vi "XY Graph Get Plots Metadata.vi"(8 "Error In":errorcluster, 11 "XYGraph Ref":T1) -> (0 "Error Out":errorcluster, 1 "Plot Metadata Found?":bool, 2 "Plot Metadata":variant[](array[variant]), 3 "XYGraph Ref (dup)":T1)   [LabVIEW 2021, in "XY Graph Add-Ons.lvlib"]
uses:
  XY Graph Add-Ons.lvlib
  XY Graph Refnum.ctl
  XY Graph Property Tag List.ctl
  <vilib>/UserTags/UserTags.lvlib
panel:
  # "see the License on the block diagram (Ctrl+E or Window:Show Block Diagram)"
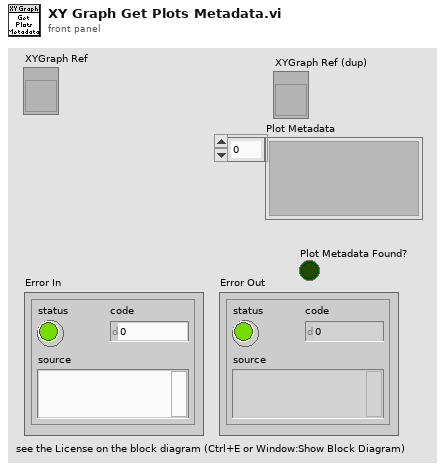
[diagram p1: front panel]
types:
  T1 = typedef "XY Graph Add-Ons.lvlib/XY Graph Refnum.ctl" = refnum<vi>
  T2 = typedef "XY Graph Add-Ons.lvlib/XY Graph Property Tag List.ctl" = enum16{"Max Legend Size", "Preserved Plots", "XScales.GridColors", "YScales.GridColors", "TipStrip String", "TipStrip Visible", "Tool Panels Visibility", "Plot Metadata"}
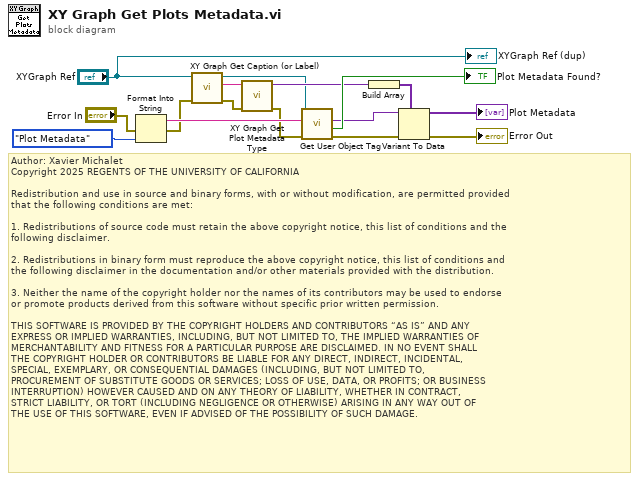
[diagram p0: block diagram]
diagram:
  # "Author: Xavier Michalet\nCopyright 2025 REGENTS OF THE UNIVERSITY OF CALIFORNIA\n\nRedistribution and use in source and binary forms, with or without modification, are permitted provided\nthat the following conditions are met:\n\n1. Redistributions of source code must retain the above copyright notice, this list of conditions and the\nfollowing disclaimer.\n\n2. Redistributions in binary form must reproduce the above copyright notice, this list of conditions and\nthe following disclaimer in the documentation and/or other materials provided with the distribution.\n\n3. Neither the name of the copyright holder nor the names of its contributors may be used to endorse \nor promote products derived from this software without specific prior written permission.\n\nTHIS SOFTWARE IS PROVIDED BY THE COPYRIGHT HOLDERS AND CONTRIBUTORS “AS IS” AND ANY \nEXPRESS OR IMPLIED WARRANTIES, INCLUDING, BUT NOT LIMITED TO, THE IMPLIED WARRANTIES OF\nMERCHANTABILITY AND FITNESS FOR A PARTICULAR PURPOSE ARE DISCLAIMED. IN NO EVENT SHALL\nTHE COPYRIGHT HOLDER OR CONTRIBUTORS BE LIABLE FOR ANY DIRECT, INDIRECT, INCIDENTAL, \nSPECIAL, EXEMPLARY, OR CONSEQUENTIAL DAMAGES (INCLUDING, BUT NOT LIMITED TO, \nPROCUREMENT OF SUBSTITUTE GOODS OR SERVICES; LOSS OF USE, DATA, OR PROFITS; OR BUSINESS\nINTERRUPTION) HOWEVER CAUSED AND ON ANY THEORY OF LIABILITY, WHETHER IN CONTRACT, \nSTRICT LIABILITY, OR TORT (INCLUDING NEGLIGENCE OR OTHERWISE) ARISING IN ANY WAY OUT OF\nTHE USE OF THIS SOFTWARE, EVEN IF ADVISED OF THE POSSIBILITY OF SUCH DAMAGE."
  n1 = Format Into String(error in="Error In", XY_Graph_Property_Tag_List."Plot Metadata" ("XY Graph Property Tag")) -> (resulting string=w14:string, error out=w4:errorcluster)  [unwired: 2 in]
  n2 = call "XY Graph Get Caption (or Label).vi"("error in (no error)"=w4, "XY Graph in"="XYGraph Ref") -> ("error out"=w3:errorcluster, "Caption (or Label) Text"=w10:string, "XY Graph out"=w6:T1)  [unwired: 7 in]
  n3 = call "XY Graph Get Plot Metadata Type.vi"("Error In"=w3, "Graph Label"=w10) -> ("Error Out"=w8:errorcluster, "Plot Metadata Type"=w9:variant)  [unwired: 7 in, 1 out]
  n4 = call <vilib>:"Get User Object Tag.vi"("error in (no error)"=w8, "Tag Name"=w14, "Generic Refnum"=w6) -> ("error out"=w12:errorcluster, "Was Tag Found?"=→"Plot Metadata Found?":bool, "Value"=w13:variant)  [unwired: 5 in, 1 out]
  n5 = Build Array(w9) -> (w7:variant[])
  n6 = Variant To Data(error in=w12, type=w7, Variant=w13) -> (data=→"Plot Metadata":variant[], error out=→"Error Out":errorcluster)
  "XYGraph Ref (dup)" <- "XYGraph Ref"
